vi "Application Refnum.vi"() -> ()   [LabVIEW 2017, in "Assertion.Tests.lvlib" / "Assert Refnum.lvlib"]
uses:
  Assert Refnum.lvlib
  Assertion/Assertion.lvlib
panel:
  out "error out":errorcluster
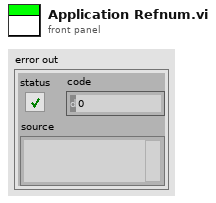
[diagram p1: front panel]
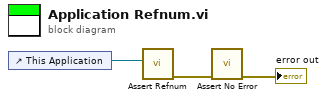
[diagram p0: block diagram]
diagram:
  n1 = control-ref of="This Application"() -> (w1:refnum<vi>)
  n2 = call "Assert Refnum.vi"("Refnum"=w1) -> ("error out"=w3:errorcluster)  [unwired: 10 in]
  n3 = call "Assert No Error.vi"("error in (no error)"=w3) -> ("error out"=→"error out":errorcluster)  [unwired: 10 in]
